vi "Large integer U8 array - more than 0.vi"(5 "Large number - U8":T1) -> (1 "> 0 ?":bool)   [LabVIEW 2013]
doc: "If any element in a large numbers (U8 array format) is not zero returns true."
uses:
  User Access Type defs/Large number - U8 array.ctl
panel:
  # "index 0 = LSD"
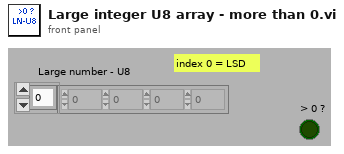
[diagram p1: front panel]
types:
  T1 = typedef "Large number - U8 array.ctl" = u8[]
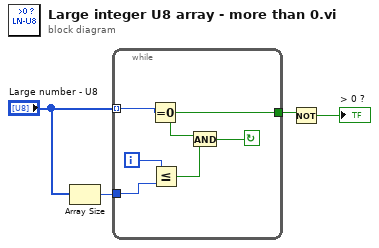
[diagram p0: block diagram]
diagram:
  n1 = Array Size(array="Large number - U8") -> (size(s)=w3:i32)
  n2 = while {
    tunnel: "Large number - U8" -> [w10] mode=indexing
    tunnel: w3 -> [w7]
    tunnel: [w9] -> w2
    i -> [w8]
    stop <- w5 continue-if-true
    n3 = Equal To 0?(x=w10) -> (x = 0?=w9:bool)
    n4 = Less Or Equal?(x=w8, y=w7) -> (x <= y?=w6:bool)
    n5 = And(x=w9, y=w6) -> (x .and. y?=w5:bool)
  }
  n6 = Not(x=w2) -> (.not. x?=→"> 0 ?":bool)
